vi "pthread_mutex_trylock.vi"(8 "error in (no error)":errorcluster, 11 "mutex ptr in":u64) -> (0 "error out":errorcluster, 2 "lock success?":bool, 3 "mutex ptr out":u64)   [LabVIEW 2016, in "Linux RT IPC.POSIX Threads.lvlib" / "POSIX Thread Object.lvclass"]
uses:
  POSIX Thread Object.lvclass
  Controls/pthread functions.ctl
  <vilib>/NI/NI Linux RT Errno/Controls/Public/errno.ctl
  <vilib>/NI/NI Linux RT Errno/Linux Errno.lvlib
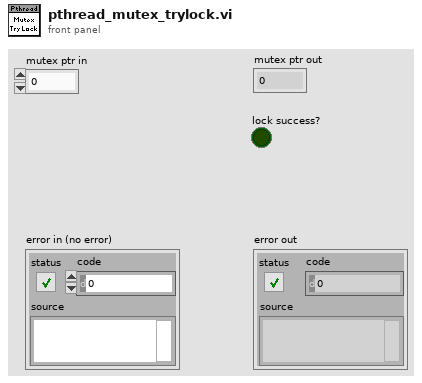
[diagram p1: front panel]
types:
  T1 = typedef "Linux Errno.lvlib/errno.ctl" = enum16{"NO ERROR", "EPERM", "ENOENT", "ESRCH", "EINTR", "EIO", "ENXIO", "E2BIG", "ENOEXEC", "EBADF", "ECHILD", "EAGAIN", "ENOMEM", "EACCES", "EFAULT", "ENOTBLK", "EBUSY", "EEXIST", "EXDEV", "ENODEV", "ENOTDIR", "EISDIR", "EINVAL", "ENFILE", "EMFILE", "ENOTTY", "ETXTBSY", "EFBIG", "ENOSPC", "ESPIPE", "EROFS", "EMLINK", "EPIPE", "EDOM", "ERANGE", "EDADLK", "ENAMETOOLONG", "ENOLCK", "ENOSYS", "ENOTEMPTY", "ELOOP", "EWOULDBLOCK", "ENOMSG", "EIDRM", "ECHRNG", "EL2NSYNC", "EL3HLT", "EL3RST", "ELNRNG", "EUNATCH", "ENOCSI", "EL2HLT", "EBADE", "EBADR", "EXFULL", "ENOANO", "EBADRQC", "EBADSLT", "EDEADLOCK", "EBFONT", "ENOSTR", "ENODATA", "ETIME", "ENOSR", "ENONET", "ENOPKG", "EREMOTE", "ENOLINK", "EADV", "ESRMNT", "ECOMM", "EPROTO", "EMULTIHOP", "EDOTDOT", "EBADMSG", "EOVERFLOW", "ENOTUNIQ", "EBADFD", "EREMCHG", "ELIBACC", "ELIBBAD", "ELIBSCN", "ELIBMAX", "ELIBEXEC", "ELISEQ", "ERESTART", "ESTRPIPE", "EUSERS", "ENOTSOCK", "EDESTADDRREQ", "EMSGSIZE", "EPROTOTYPE", "ENOPROTOOPT", "EPROTONOSUPPORT", "ESOCKTNOSUPPORT", "EOPNOTSUPP", "EPFNOSUPPORT", "EAFNOSUPPORT", "EADDRINUSE", "EADDRNOTAVAIL", "ENETDOWN", "ENETUNREACH", "ENETRESET", "ECONNABORTED", "ECONNRESET", "ENOBUFS", "EISCONN", "ENOTCONN", "ESHUTDOWN", "ETOOMANYREFS", "ETIMEDOUT", "ECONNREFUSED", "EHOSTDOWN", "EHOSTUNREACH", "EALREADY", "EINPROGRESS", "ESTALE", "EUCLEAN", "ENOTNAM", "ENAVAIL", "EISNAM", "EREMOTEIO", "EDQUOT", "ENOMEDIUM", "EMEDIUMTYPE", "ECANCELED", "ENOKEY", "EKEYEXPIRED", "EKEYREVOKED", "EKEYREJECTED", "EOWNERDEAD", "ENOTRECOVERABLE", "ERFKILL", "EHWPOISON", "UNDEFINED"}
  T2 = typedef "Linux RT IPC.POSIX Threads.lvlib/POSIX Thread Object.lvclass/pthread functions.ctl" = enum16{"unspecified", "pthread_condattr_init", "pthread_condattr_destroy", "pthread_condattr_getclock", "pthread_condattr_setclock", "pthread_condattr_getpshared", "pthread_condattr_setpshared", "pthread_cond_init", "pthread_cond_destroy", "pthread_cond_broadcast", "pthread_cond_signal", "pthread_cond_timedwait", "pthread_cond_wait", "pthread_mutexattr_init", "pthread_mutexattr_destroy", "pthread_mutexattr_getprioceiling", "pthread_mutexattr_setprioceiling", "pthread_mutexattr_getprotocol", "pthread_mutexattr_setprotocol", "pthread_mutexattr_getpshared", "pthread_mutexattr_setpshared", "pthread_mutexattr_gettype", "pthread_mutexattr_settype", "pthread_mutex_init", "pthread_mutex_destroy", "pthread_mutex_getprioceiling", "pthread_mutex_setprioceiling", "pthread_mutex_lock", "pthread_mutex_timedlock", "pthread_mutex_trylock", "pthread_mutex_unlock", "sem_destroy", "sem_getvalue", "sem_init", "sem_open", "sem_post", "sem_timedwait", "sem_trywait", "sem_wait", "barrier_init", "barrier_destroy", "barrier_wait", "barrierattr_init", "barrierattr_destroy", "barrierattr_getpshared", "barrierattr_setpshared"}
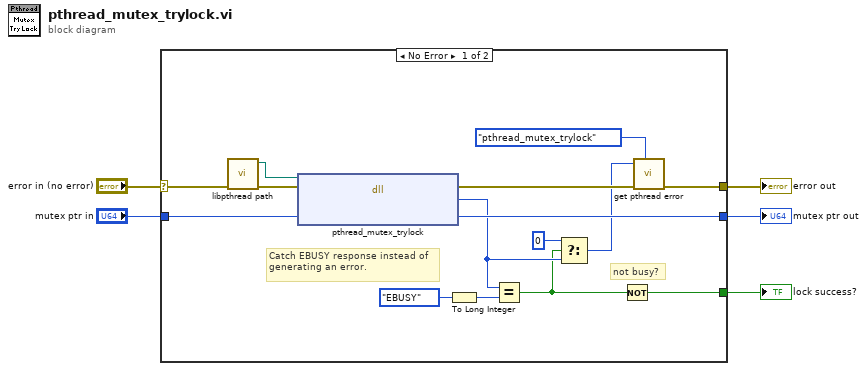
[diagram p0: block diagram]
diagram:
  n1 = case shown="No Error" "error in (no error)" {
    selector: "error in (no error)" -> [w20 w22]
    tunnel: "mutex ptr in" -> [w19 w21]
    tunnel: [w18 w22] -> w3
    tunnel: [w17 w21] -> w2
    tunnel: [w16 _] -> w1
    frame No Error {
      # "Catch EBUSY response instead of generating an error."
      # "not busy?"
      n2 = call "libpthread path.vi"("error in (no error)"=w20) -> ("error out"=w14:errorcluster, "path to libpthread"=w15:path)  [unwired: 9 in]
      n3 = dll-call lib="?" fn="pthread_mutex_trylock"(path in=w15, error in=w14, "mutex"=w19) -> (error out=w13:errorcluster, "errno"=w9:i32, "mutex"=w17:u64)  [unwired: 1 in, 1 out]
      n4 = To Long Integer(number=errno."EBUSY" ("errno")) -> (32bit integer=w11:i32)
      n5 = Equal?(x=w9, y=w11) -> (x = y?=w7:bool)
      n6 = Select(t=0, s=w7, f=w9) -> (s? t:f=w10:i32)
      n7 = Not(x=w7) -> (.not. x?=w16:bool)
      n8 = call "get pthread error.vi"("function"=pthread_functions."pthread_mutex_trylock", "error in (no error)"=w13, "errno"=w10) -> ("error out"=w18:errorcluster)  [unwired: 8 in]
    }
    frame Error {
    }
  }
  "error out" <- w3
  "mutex ptr out" <- w2
  "lock success?" <- w1
